vi "UTIL Generate Analog Output_Final.vi"(6 "sampling info":cluster{"Fs":dbl, "#s":dbl}={"Fs"=1000.0, "#s"=1000.0} {"Fs" format="%.2p"}, 8 "error in (no error)":errorcluster, 9 "frequency":dbl=10.0 format="%0.2p", 10 "amplitude":dbl=1.0 format="%0.2p", 11 "task/channels in":refnum<k21>) -> (0 "error out":errorcluster, 3 "task out":refnum<k21>)   [LabVIEW 2017]
uses:
  <vilib>/DAQmx/write.llb/DAQmx Write (Analog Wfm 1Chan NSamp).vi
  <vilib>/DAQmx/miscellaneous.llb/DAQmx Fill In Error Info.vi
  <vilib>/measure/NI_MABase.lvlib
panel:
  in  "stop":bool
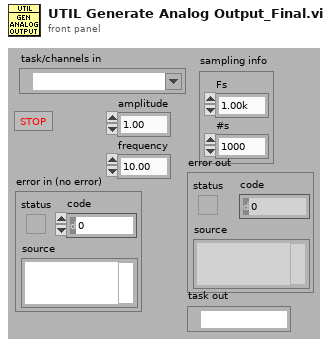
[diagram p1: front panel]
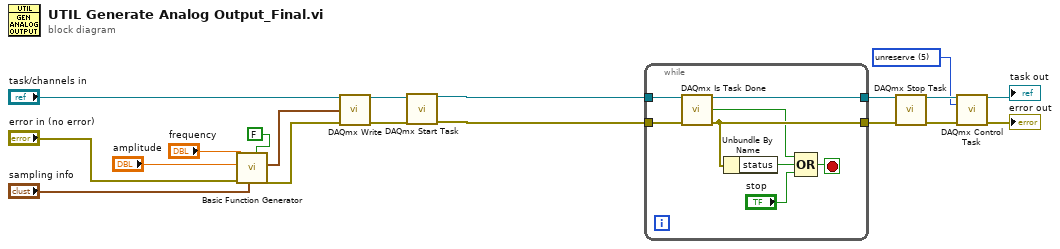
[diagram p0: block diagram]
diagram:
  w1 = 5 items=["verify"=2, "reserve"=4, "commit"=3, "unreserve"=5, "abort"=6] ("action")
  n1 = call <vilib>:"Basic Function Generator.vi"("reset signal"=FALSE, "sampling info"="sampling info", "error in (no error)"="error in (no error)", "amplitude"="amplitude", "frequency"="frequency") -> ("error out"=w16:errorcluster, "signal out"=w15:waveform(dbl))  [unwired: 4 in, 1 out]
  n2 = call-poly <vilib>:"DAQmx Write.vi"("task/channels in"="task/channels in", "data"=w15, "error in"=w16) -> ("task out"=w13:refnum<k21>, "error out"=w14:errorcluster)  [unwired: 10 in, 1 out]
  n3 = call <vilib>:"DAQmx Start Task.vi"("task/channels in"=w13, "error in"=w14) -> ("task out"=w7:refnum<k21>, "error out"=w6:errorcluster)  [unwired: 12 in]
  n4 = while {
    tunnel: [w27] -> w9
    tunnel: [w26] -> w8
    tunnel: w7 -> [w21]
    tunnel: w6 -> [w20]
    stop <- w22 stop-if-true
    n5 = call <vilib>:"DAQmx Is Task Done.vi"("task/channels in"=w21, "error in"=w20) -> ("task out"=w27:refnum<k21>, "task done?"=w23:bool, "error out"=w26:errorcluster)  [unwired: 11 in]
    n6 = Unbundle By Name(w26) -> ("status"=w24:bool)
    n7 = Compound Arithmetic op=OR(w23, w24, "stop") -> (w22:bool)
  }
  n8 = call <vilib>:"DAQmx Stop Task.vi"("task/channels in"=w9, "error in"=w8) -> ("task out"=w5:refnum<k21>, "error out"=w3:errorcluster)  [unwired: 12 in]
  n9 = call <vilib>:"DAQmx Control Task.vi"("task/channels in"=w5, "action"=w1, "error in"=w3) -> ("task out"=→"task out":refnum<k21>, "error out"=→"error out":errorcluster)  [unwired: 11 in]
